vi "PosNegNo.vi"(9 "String 2":string, 10 "A":dbl, 11 "String":string) -> (3 "String 3":string)   [LabVIEW 2021]
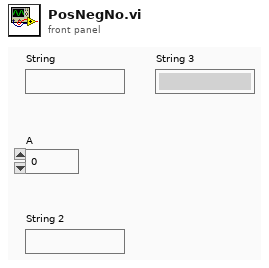
[diagram p1: front panel]
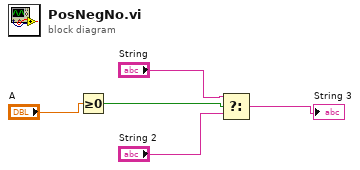
[diagram p0: block diagram]
diagram:
  n1 = Greater Or Equal To 0?(x="A") -> (x >= 0?=w3:bool)
  n2 = Select(t="String", s=w3, f="String 2") -> (s? t:f=→"String 3":string)
